vi "Setpoint temperature control.vi"(0 "Meerstetter Lib.lvlib:TEC 1090":refnum<class "Meerstetter TEC.lvclass">, 1 "Setpoint":sgl, 3 "error in":errorcluster) -> (7 "TEC 1090 out":refnum<class "Meerstetter TEC.lvclass">, 10 "error out":errorcluster)   [LabVIEW 2015, in "Meerstetter Lib.lvlib" / "Meerstetter TEC.lvclass"]
uses:
  Meerstetter TEC.lvclass
  Configurable Device/Configurable Device.lvclass/Configurable Device.ctl
  Configurable Device/Read Log Session.vi
  Configurable Device/Read ID.vi
  <vilib>/MSR Consulting, LLC/ESF/Session - Root.lvclass
  reusable/Session APIs/Session Log/System Log.lvclass
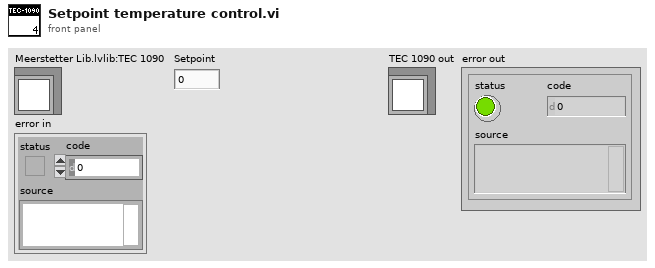
[diagram p1: front panel]
types:
  T1 = typedef "Session - Root.lvclass/Session Handle.ctl" = refnum<data-value>
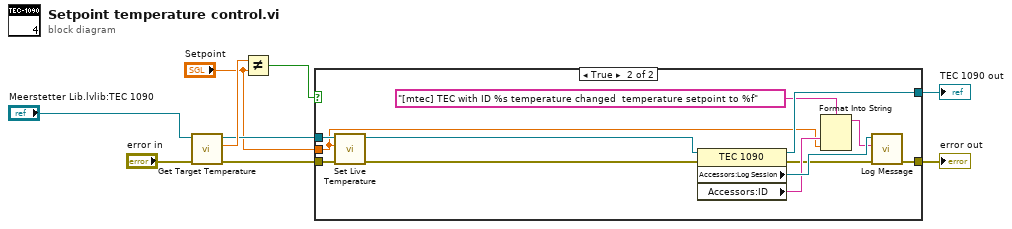
[diagram p0: block diagram]
diagram:
  n1 = call "Get Target Temperature.vi"("error in"="error in", "TEC 1090 in"="Meerstetter Lib.lvlib:TEC 1090") -> ("error out"=w5:errorcluster, "Number"=w8:sgl, "TEC 1090 out"=w7:refnum<class "Meerstetter TEC.lvclass">)  [unwired: 7 in]
  n2 = Not Equal?(x=w8, y="Setpoint") -> (x != y?=w1:bool)
  n3 = case shown="True" w1 {
    tunnel: w7 -> [w11 w19]
    tunnel: [w11 w20] -> w4
    tunnel: w5 -> [w10 w23]
    tunnel: [w10 w12] -> w3
    tunnel: "Setpoint" -> [_ w16]
    frame False {
    }
    frame True {
      n4 = call "Set Live Temperature.vi"("error in"=w23, "T"=w16, "TEC 1090 in"=w19) -> ("error out"=w14:errorcluster, "TEC 1090 out"=w21:refnum<class "Meerstetter TEC.lvclass">)  [unwired: 7 in]
      n5 = property class="TEC 1090"(reference=w21, error in=w14) -> (reference out=w20:refnum<class "Meerstetter TEC.lvclass">, error out=w13:errorcluster, "Accessors:Log Session"=w22:T1, "Accessors:ID"=w17:string)
      n6 = Format Into String(format string="[mtec] TEC with ID %s temperature changed  temperature setpoint to %f", w17, w16) -> (resulting string=w15:string)  [unwired: 2 in, 1 out]
      n7 = call "Log Message.vi"("error in"=w13, "MSG In"=w15, "session in"=w22) -> ("error out"=w12:errorcluster)  [unwired: 7 in, 1 out]
    }
  }
  "TEC 1090 out" <- w4
  "error out" <- w3
